vi "Max Min Value.vi"(9 "ZArray":dbl[](array[numeric]), 10 "YArray":dbl[](array[numeric]), 11 "XArray":dbl[](array[numeric])) -> (1 "MaxValue":dbl, 2 "output cluster":T1, 3 "array":dbl[](array[numeric]))   [LabVIEW 2011]
panel:
  in  "input cluster 2":cluster{"X-mag":dbl, "Y-mag":dbl, "Z-mag":dbl}
  in  "input cluster":T1
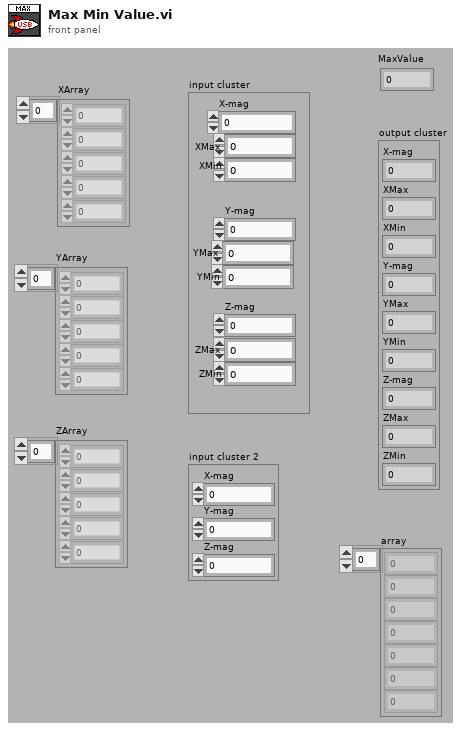
[diagram p1: front panel]
types:
  T1 = cluster{"X-mag":dbl, "XMax":dbl, "XMin":dbl, "Y-mag":dbl, "YMax":dbl, "YMin":dbl, "Z-mag":dbl, "ZMax":dbl, "ZMin":dbl}
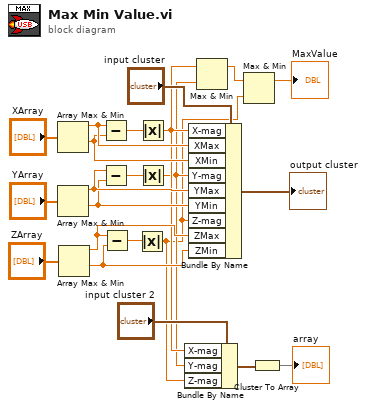
[diagram p0: block diagram]
diagram:
  n1 = Array Max & Min(array="XArray") -> (max value=w17:dbl, min value=w16:dbl)  [unwired: 2 out]
  n2 = Array Max & Min(array="YArray") -> (max value=w15:dbl, min value=w14:dbl)  [unwired: 2 out]
  n3 = Array Max & Min(array="ZArray") -> (max value=w11:dbl, min value=w10:dbl)  [unwired: 2 out]
  n4 = Subtract(x=w17, y=w16) -> (x-y=w21:dbl)
  n5 = Subtract(x=w15, y=w14) -> (x-y=w22:dbl)
  n6 = Subtract(x=w11, y=w10) -> (x-y=w12:dbl)
  n7 = Absolute Value(x=w12) -> (abs(x)=w3:dbl)
  n8 = Absolute Value(x=w21) -> (abs(x)=w5:dbl)
  n9 = Absolute Value(x=w22) -> (abs(x)=w4:dbl)
  n10 = Bundle By Name(cluster="input cluster 2", "X-mag"=w5, "Y-mag"=w4, "Z-mag"=w3) -> (w2:cluster{"X-mag":dbl, "Y-mag":dbl, "Z-mag":dbl})
  n11 = Bundle By Name(cluster="input cluster", "X-mag"=w5, "XMax"=w17, "XMin"=w16, "Y-mag"=w4, "YMax"=w15, "YMin"=w14, "Z-mag"=w3, "ZMax"=w11, "ZMin"=w10) -> (→"output cluster":T1)
  n12 = Max & Min(x=w5, y=w4) -> (max(x,y)=w9:dbl)  [unwired: 1 out]
  n13 = Max & Min(x=w9, y=w3) -> (max(x,y)=→"MaxValue":dbl)  [unwired: 1 out]
  n14 = Cluster To Array(cluster=w2) -> (array=→"array":dbl[])
